vi "Evaluate Part 2.vi"() -> ()   [LabVIEW 2021]
uses:
  Proto/xmas.ctl
  Proto/Rule.lvclass
panel:
  out "sum":u64
  in  "Input":string="px{a<2006:qkq,m>2090:A,rfg}\npv{a>1716:R,A}\nlnx{m>1548:A,A}\nrfg{s<537:gd,x>2440:R,A}\nqs{s>3448:A,lnx}\nqkq{x<1416:A,crn}\ncrn{x>2662:A,R}\nin{s<1351:px,qqz}\nqqz{s>2770:qs,m<1801:hdj,R}\ngd{a>3333:R,R}\nhdj{m>838:A,pv}\n\n{x=787,m=2655,a=1222,s=2876}\n{x=1679,m=44,a=2067,s=496}\n{x=2036,m=264,a=79,s=2244}\n{x=2461,m=1339,a=466,s=291}\n{x=2127,m=1623,a=2188,s=1013}"
  # "167409079868000"
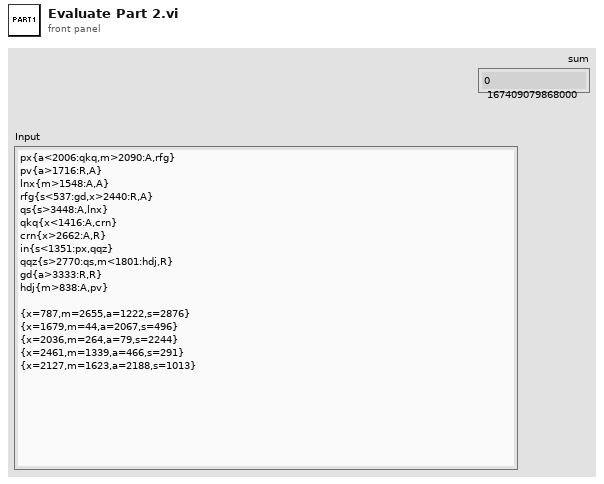
[diagram p1: front panel]
types:
  T1 = typedef "xmas.ctl" = cluster{"from":cluster{"x":u64, "m":u64, "a":u64, "s":u64}, "to":cluster{"x":u64, "m":u64, "a":u64, "s":u64}}
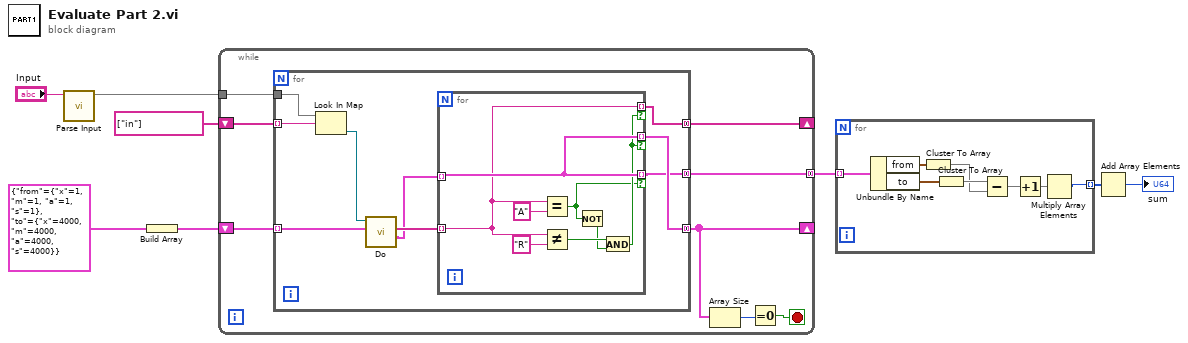
[diagram p0: block diagram]
diagram:
  n1 = call "Parse Input.vi"("Input"="Input") -> ("map"=w7:map{string, refnum<class "Rule.lvclass">})  [unwired: 9 in, 1 out]
  n2 = Build Array(T1 {"from"={"x"=1, "m"=1, "a"=1, "s"=1}, "to"={"x"=4000, "m"=4000, "a"=4000, "s"=4000}} ("In Range")) -> (w5:T1[])
  n3 = while {
    shift-right: [w13] -> _
    shift-left: string[] ["in"] ("key") -> [w16]
    tunnel: w7 -> [w15]
    shift-right: [w11] -> _
    shift-left: w5 -> [w14]
    tunnel: [w12] -> w3 mode=concatenating
    stop <- w9 stop-if-true
    n4 = for {
      tunnel: w16 -> [w25] mode=indexing
      tunnel: w15 -> [w24]
      tunnel: w14 -> [w21] mode=indexing
      tunnel: [w19] -> w13 mode=concatenating
      tunnel: [w18] -> w11 mode=concatenating
      tunnel: [w17] -> w12 mode=concatenating
      n5 = Look In Map(map=w24, key=w25) -> (value=w23:refnum<class "Rule.lvclass">)  [unwired: 1 in, 1 out]
      n6 = call "Do.vi"("In Range"=w21, "Rule In"=w23) -> ("Out Range"=w20:T1[], "Label"=w22:string[])  [unwired: 6 in, 2 out]
      n7 = for {
        tunnel: w22 -> [w30] mode=indexing
        tunnel: w20 -> [w31] mode=indexing
        tunnel: [w31] -> w17 mode=indexing if=w27
        tunnel: [w31] -> w18 mode=indexing if=w28
        tunnel: [w30] -> w19 mode=indexing if=w28
        n8 = Equal?(x=w30, y="A") -> (x = y?=w27:bool)
        n9 = Not Equal?(x=w30, y="R") -> (x != y?=w29:bool)
        n10 = Not(x=w27) -> (.not. x?=w26:bool)
        n11 = And(x=w29, y=w26) -> (x .and. y?=w28:bool)
      }
    }
    n12 = Array Size(array=w11) -> (size(s)=w10:i32)
    n13 = Equal To 0?(x=w10) -> (x = 0?=w9:bool)
  }
  n14 = for {
    tunnel: w3 -> [w41] mode=indexing
    tunnel: [w34] -> w1 mode=indexing
    n15 = Unbundle By Name(w41) -> ("from"=w40:cluster{"x":u64, "m":u64, "a":u64, "s":u64}, "to"=w39:cluster{"x":u64, "m":u64, "a":u64, "s":u64})
    n16 = Cluster To Array(cluster=w40) -> (array=w37:u64[])
    n17 = Cluster To Array(cluster=w39) -> (array=w38:u64[])
    n18 = Subtract(x=w38, y=w37) -> (x-y=w36:u64[])
    n19 = Increment(x=w36) -> (x+1=w35:u64[])
    n20 = Multiply Array Elements(1:w35) -> (0:w34:u64)
  }
  n21 = Add Array Elements(numeric array=w1) -> (sum=→"sum":u64)
